vi "Write ISO Format.vi"(10 "ISO Format":T1, 11 "DateTime.ISO8601 in":refnum<class "DateTime.ISO8601.lvclass">) -> (3 "DateTime.ISO8601 out":refnum<class "DateTime.ISO8601.lvclass">)   [LabVIEW 2018, in "DateTime.ISO8601.lvclass"]
uses:
  DateTime.ISO8601.lvclass
  ISO8601 Date Formats.ctl
  DateTime.ISO8601.lvclass/DateTime.ISO8601.ctl
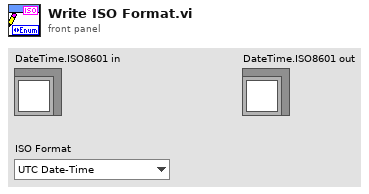
[diagram p1: front panel]
types:
  T1 = typedef "ISO8601 Date Formats.ctl" = enum16{"UTC Date-Time", "Date", "Calendar Month", "Week", "Week-Day", "Month-Day", "Ordinal Date"}
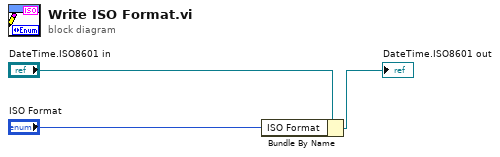
[diagram p0: block diagram]
diagram:
  n1 = Bundle By Name(cluster="DateTime.ISO8601 in", "ISO Format"="ISO Format") -> (→"DateTime.ISO8601 out":refnum<class "DateTime.ISO8601.lvclass">)
